vi "aal_CIC (real input).vi"(1 "Reset":bool, 2 "Stages":i32, 3 "N":i32=1, 4 "x":dbl[](array[numeric])) -> (0 "y":dbl[](array[numeric]))   [LabVIEW 2020, in "NI_AALPro.lvlib"]
uses:
  NI_AALPro.lvlib
  aal_moving average with decimation by order (real input).vi
  aal_cascaded moving average (real input).vi
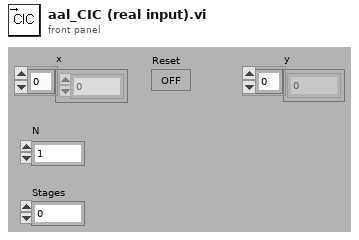
[diagram p1: front panel]
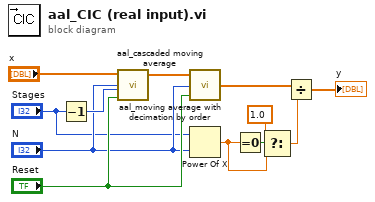
[diagram p0: block diagram]
diagram:
  n1 = Decrement(x="Stages") -> (x-1=w12:i32)
  n2 = call-poly "aal_cascaded moving average.vi"("Reset"="Reset", "Stages"=w12, "N"="N", "x"="x") -> ("y"=w11:dbl[])
  n3 = call-poly "aal_moving average with decimation by order.vi"("Reset"="Reset", "N"="N", "x"=w11) -> ("y"=w9:dbl[])
  n4 = Power Of X(1:"N", 2:"Stages") -> (0:w3:dbl)
  n5 = Equal To 0?(x=w3) -> (x = 0?=w6:bool)
  n6 = Select(t=1.0, s=w6, f=w3) -> (s? t:f=w5:dbl)
  n7 = Divide(x=w9, y=w5) -> (x/y=→"y":dbl[])
